vi "Yokogawa WT300 Series Measure Continuous Normal.vi"() -> ()   [LabVIEW 2016]
doc: "This example shows how to measure the normal numeric data continuously."
uses:
  Public/Utility/Function/Create Function String (Harmonics).vi
  Public/Data/Read Measurement (Normal).vi
  Yokogawa WT300 Series.lvlib
panel:
  in  "Function (0: Uthd)":i32(ring) items=["Uthd", "Ithd"]
  in  "Element (1: 1)":i32(ring)=1 items=["1"=1, "2"=2, "3"=3, "Sigma A"=4]
  in  "Update Rate (500 ms)":dbl(ring)=0.5 items=["100m"=0.1, "250m"=0.25, "500m"=0.5, "1"=1.0, "2"=2.0, "5"=5.0]
  in  "Stop":bool
  out "Function":string
  out "Measurement":dbl
  in  "Item (1)":i32=1 min=1 max=255 step=1
  in  "Timeout (10000 ms)":i32=10000 min=1
  in  "VISA resource name":refnum<visa-resource-name>
  # "(c) 2013 Yokogawa Meters & Instruments Corporation.  All rights reserved."
  # "WT300 SERIES POWER ANALYZER"
  # "s"
  # "ms"
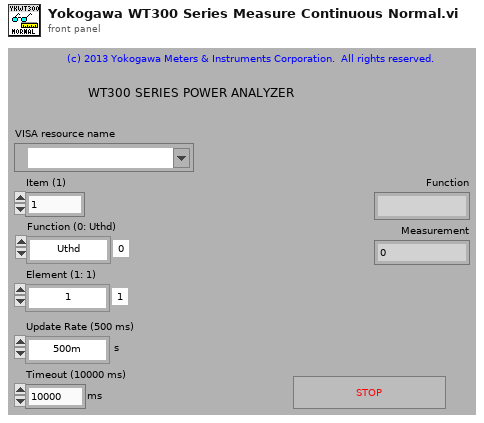
[diagram p1: front panel]
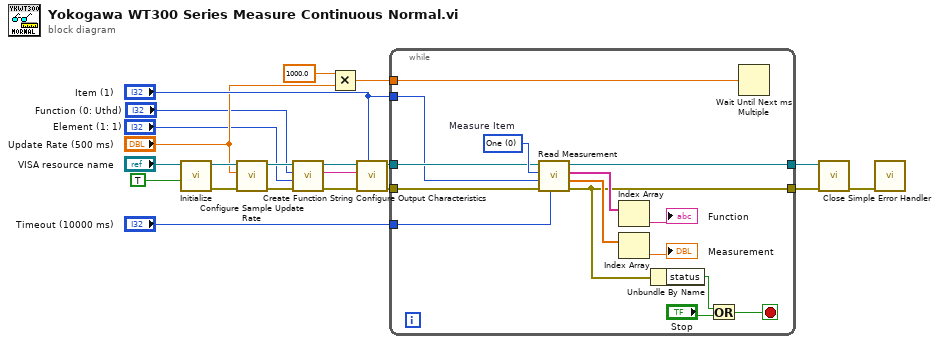
[diagram p0: block diagram]
diagram:
  n1 = call "Initialize.vi"("Reset (True)"=TRUE ("Reset? (True)"), "VISA resource name"="VISA resource name") -> ("error out"=w7:errorcluster, "VISA resource name out"=w9:refnum<visa-resource-name>)  [unwired: 7 in, 1 out]
  n2 = call "Configure Sample Update Rate.vi"("error in (no error)"=w7, "Update Rate (500m s)"="Update Rate (500 ms)", "VISA resource name"=w9) -> ("error out"=w6:errorcluster, "VISA resource name out"=w8:refnum<visa-resource-name>)  [unwired: 7 in]
  n3 = call-poly "Create Function String.vi"("error in (no error)"=w6, "Element (1: 1)"="Element (1: 1)", "Function (0: Uthd)"="Function (0: Uthd)", "VISA resource name"=w8) -> ("error out"=w12:errorcluster, "Function String"=w14:string, "VISA resource name out"=w13:refnum<visa-resource-name>)  [unwired: 5 in]
  n4 = Multiply(x=1000.0, y="Update Rate (500 ms)") -> (x*y=w4:dbl)
  n5 = call "Configure Output Characteristics.vi"("Item (1)"="Item (1)", "error in (no error)"=w12, "Function (Empty)"=w14, "VISA resource name"=w13) -> ("error out"=w15:errorcluster, "VISA resource name out"=w16:refnum<visa-resource-name>)  [unwired: 6 in]
  n6 = while {
    tunnel: [w36] -> w19
    tunnel: [w23] -> w18
    tunnel: "Timeout (10000 ms)" -> [w35]
    tunnel: w16 -> [w33]
    tunnel: w15 -> [w32]
    tunnel: "Item (1)" -> [w31]
    tunnel: w4 -> [w22]
    stop <- w24 stop-if-true
    w34 = 0 items=["One", "Plural"]  # Measure Item
    n7 = call-poly "Read Measurement.vi"("Timeout (10000 ms)"=w35, "error in (no error)"=w32, "Number of Item (15)"=w31, "Measure Item (1: Plural)"=w34, "VISA resource name"=w33) -> ("error out"=w23:errorcluster, "Measurement"=w27:dbl[], "Function"=w28:string[], "VISA resource name out"=w36:refnum<visa-resource-name>)  [unwired: 3 in]
    n8 = Index Array(array=w28) -> (element=→"Function":string)  [unwired: 1 in]
    n9 = Index Array(array=w27) -> (element=→"Measurement":dbl)  [unwired: 1 in]
    n10 = Unbundle By Name ("名前でバンドル解除")(w23) -> ("status"=w25:bool)
    n11 = Or(x=w25, y="Stop") -> (x .or. y?=w24:bool)
    n12 = Wait Until Next ms Multiple(millisecond multiple=w22) -> ()  [unwired: 1 out]
  }
  n13 = call "Close.vi"("error in (no error)"=w18, "VISA resource name"=w19) -> ("error out"=w21:errorcluster)  [unwired: 9 in]
  n14 = call <vilib>:"Simple Error Handler.vi"("error in (no error)"=w21) -> ()  [unwired: 4 in, 5 out]
